vi "DMM_GUI Server.vi"(8 "error in (no error)":errorcluster, 11 "PXIe-4071 in":refnum<class "PXIe-4071.lvclass">) -> (0 "error out":errorcluster, 3 "PXIe-4071 out":refnum<class "PXIe-4071.lvclass">)   [LabVIEW 2018, in "PXIe-4071.lvclass"]
uses:
  PXIe-4071.lvclass
  PXIe-4071.lvclass/PXIe-4071.ctl
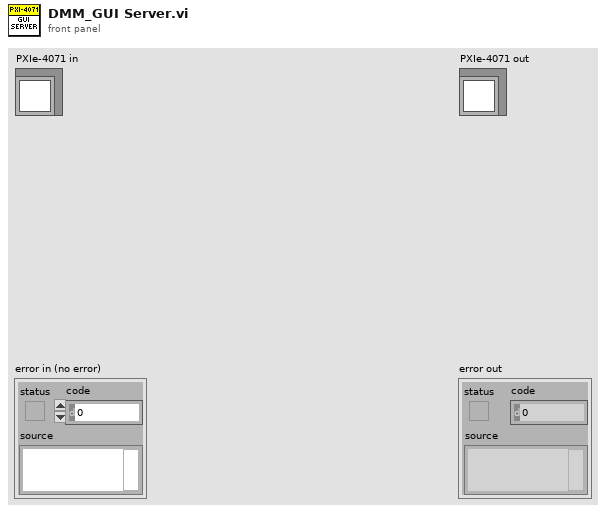
[diagram p1: front panel]
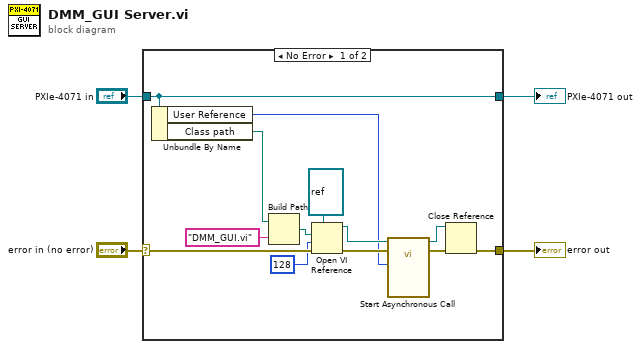
[diagram p0: block diagram]
diagram:
  n1 = case shown="No Error" "error in (no error)" {
    selector: "error in (no error)" -> [w17 w19]
    tunnel: [w13 w19] -> w3
    tunnel: [w16 w18] -> w1
    tunnel: "PXIe-4071 in" -> [w16 w18]
    frame No Error {
      n2 = Unbundle By Name(w16) -> ("User Reference"=w5:i32, "Class path"=w6:path)
      n3 = Build Path(base path=w6, name or relative path="DMM_GUI.vi") -> (appended path=w14:path)
      n4 = Open VI Reference(type specifier VI Refnum (for type only)=refnum<vi> refnum, vi path=w14, options=128, error in (no error)=w17) -> (vi reference=w7:refnum<vi>, error out=w8:errorcluster)  [unwired: 2 in]
      n5 = call-by-ref "Start Asynchronous Call"(reference=w7, error in=w8, "Instrument Reference"=w5) -> (reference out=w10:refnum<vi>, error out=w11:errorcluster)  [unwired: 10 in, 1 out]
      n6 = Close Reference(reference=w10, error in (no error)=w11) -> (error out=w13:errorcluster)
    }
    frame Error {
    }
  }
  "error out" <- w3
  "PXIe-4071 out" <- w1
